vi "find_midpoint_laser.vi"(1 "input":bool, 2 "run_time":fxp<+,40,40>) -> (0 "timeOfMidpoint":fxp<+,41,40>)   [LabVIEW 2018]
uses:
  <vilib>/rvi/FXPMathLib/FxpAdd/XNode/nifxpmath_Add.xnode
  <vilib>/rvi/FXPMathLib/FxpMul/XNode/nifxpmath_Multiplier.xnode
  <vilib>/rvi/FXPMathLib/sim/FxpSim.dll
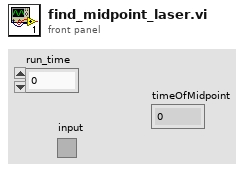
[diagram p1: front panel]
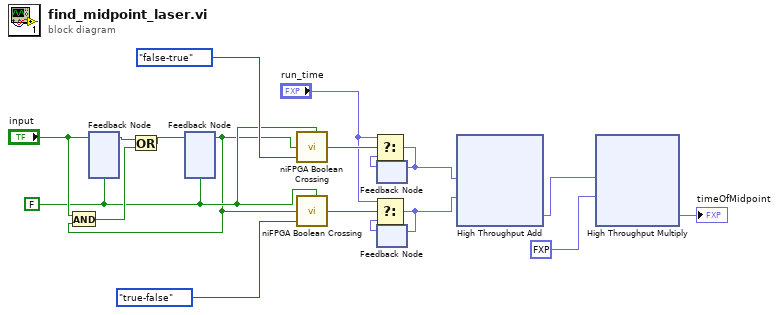
[diagram p0: block diagram]
diagram:
  w14 = FALSE
  n1 = feedback #1(w14) -> (w18:bool)
  n2 = feedback-in #1("input") -> ()
  n3 = feedback #2(w14) -> (w13:bool)
  n4 = And(x="input", y=w13) -> (x .and. y?=w16:bool)
  n5 = Or(x=w18, y=w16) -> (x .or. y?=w1:bool)
  n6 = feedback-in #2(w1) -> ()
  n7 = call <vilib>:"niFPGA Boolean Crossing.vi"("input"=w13, "direction"=enum8{"either", "false-true", "true-false"}."false-true", "initialize"=w14) -> ("crossing"=w12:bool)  [unwired: 6 in]
  n8 = call <vilib>:"niFPGA Boolean Crossing.vi"("input"=w13, "direction"=enum8{"either", "false-true", "true-false"}."true-false", "initialize"=w14) -> ("crossing"=w11:bool)  [unwired: 6 in]
  n9 = feedback #3() -> (w9:fxp<+,40,40>)  [unwired: 1 in]
  n10 = Select(t="run_time", s=w12, f=w9) -> (s? t:f=w6:fxp<+,40,40>)
  n11 = feedback-in #3(w6) -> ()
  n12 = feedback #4() -> (w10:fxp<+,40,40>)  [unwired: 1 in]
  n13 = Select(t="run_time", s=w11, f=w10) -> (s? t:f=w5:fxp<+,40,40>)
  n14 = feedback-in #4(w5) -> ()
  n15 = xnode "High Throughput Add"("x"=w6, "y"=w5) -> ("x+y"=w4:fxp<+,41,41>)
  n16 = xnode "High Throughput Multiply"("x"=w4, "y"=fxp<+,1,0> 0.5) -> ("x*y"=→"timeOfMidpoint":fxp<+,41,40>)
